vi "Day3-2.vi"() -> ()   [LabVIEW 2021]
uses:
  4dc82ad0-fb53-4f6a-a4e6-d2b65f196e0f.vi
  4388517f-81a0-45b3-bc94-ff78f6c9caee.vi
  9e6a0816-a0d4-4313-a200-a3b51abc5ec2.vi
panel:
  out "sum":i32
  out "Array":i32[](array[numeric])
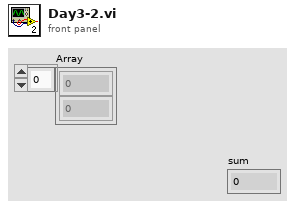
[diagram p1: front panel]
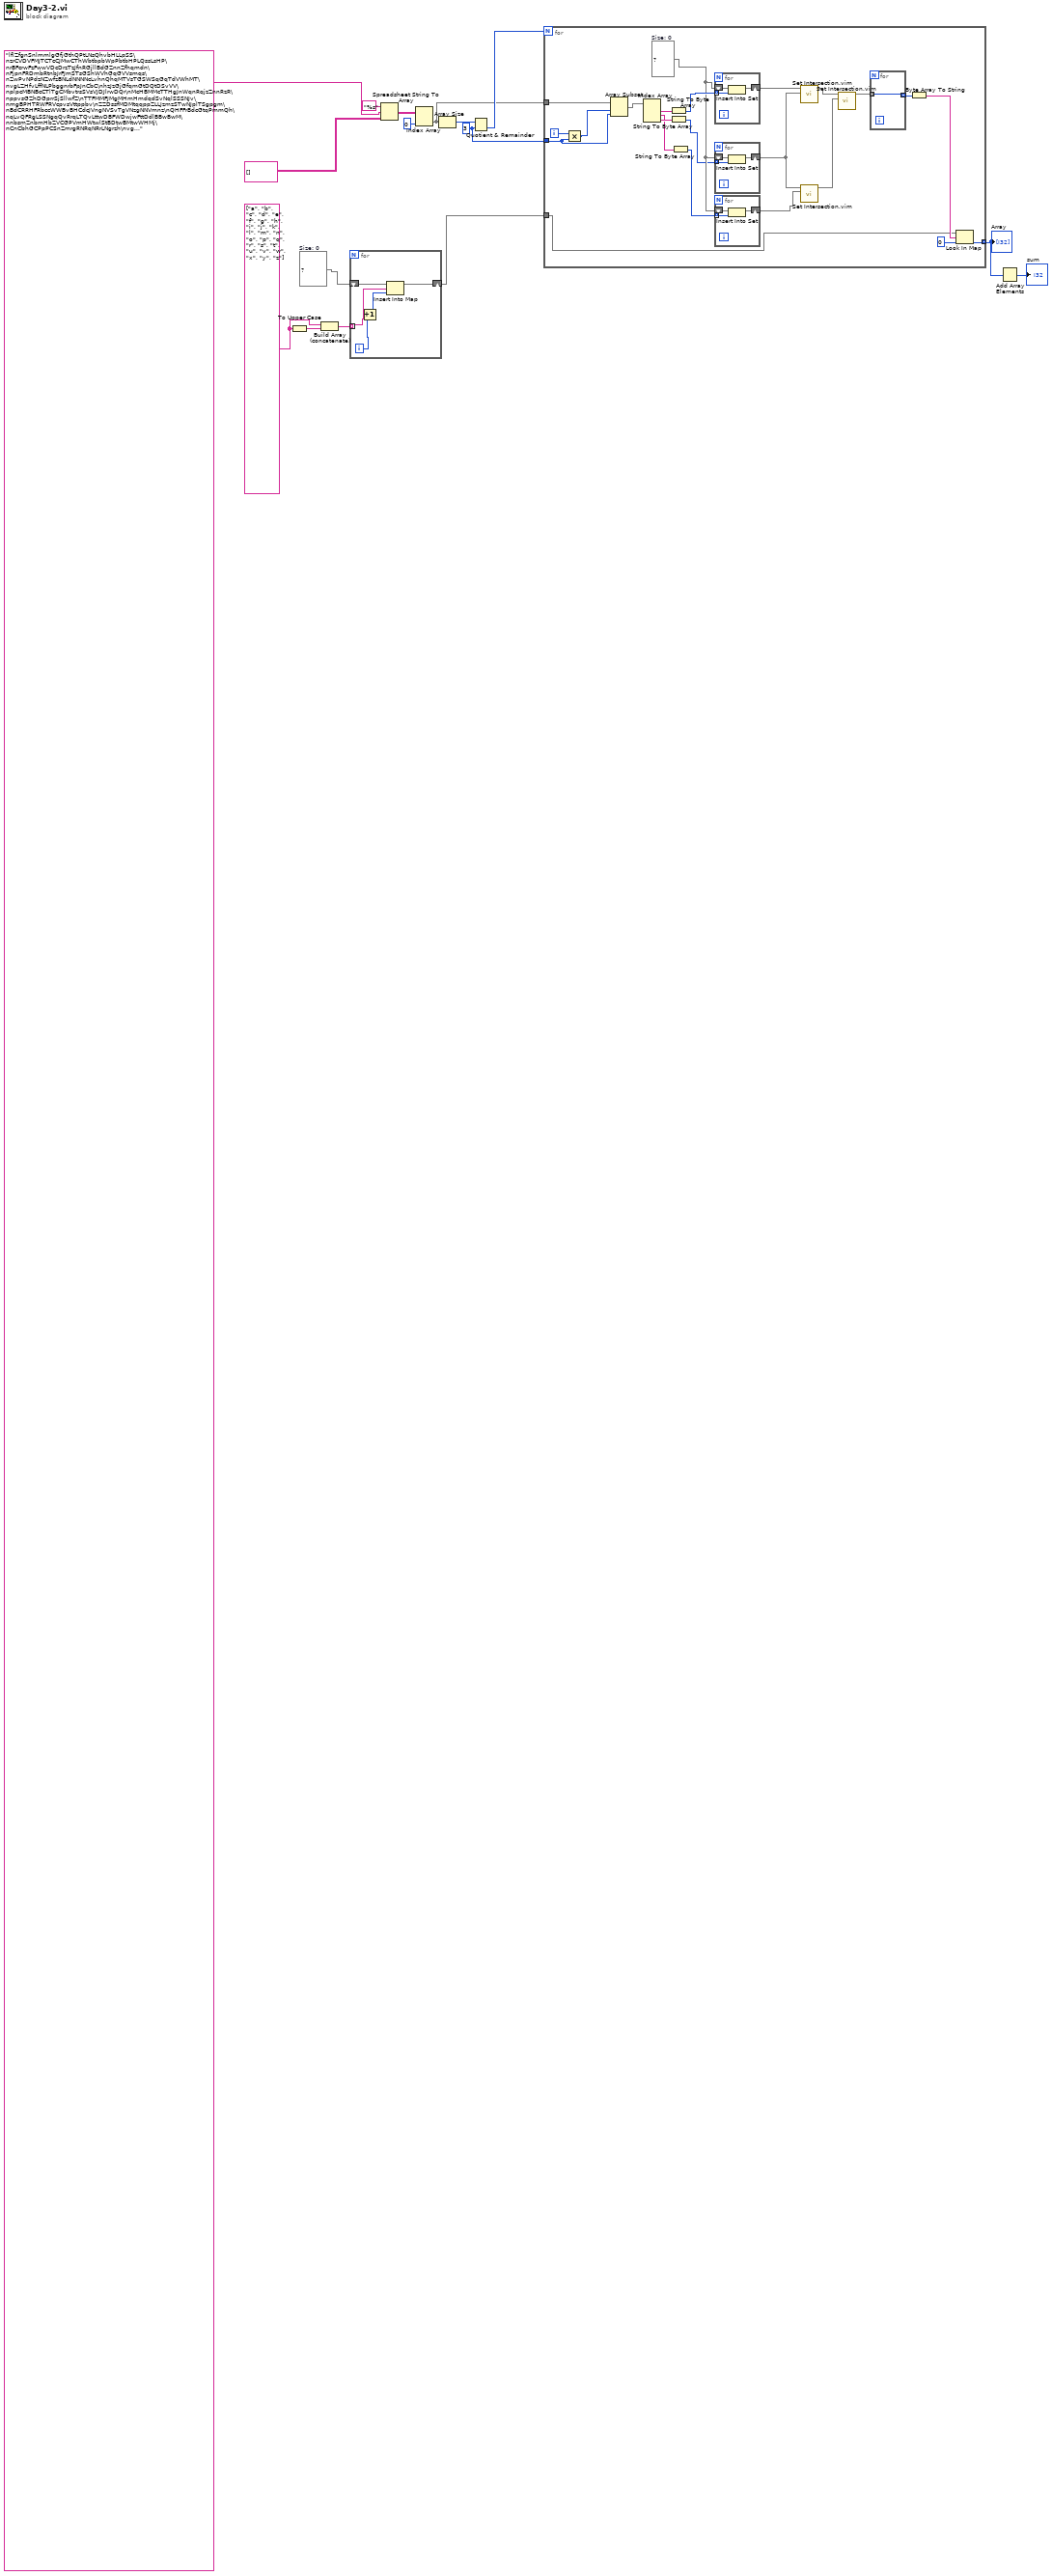
[diagram p0: block diagram]
diagram:
  w4 = 3 ("y")
  w8 = map{string, i32} {}  # Size: 0
  w10 = string[] ["a", "b", "c", "d", "e", "f", "g", "h", "i", "j", "k", "l", "m", "n", "o", "p", "q", "r", "s", "t", "u", "v", "w", "x", "y", "z"]
  n1 = To Upper Case(1:w10) -> (0:w11:string[])
  n2 = Build Array (concatenate)(w10, w11) -> (w9:string[])
  n3 = for {
    tunnel: w9 -> [w20] mode=indexing
    shift-right: [w17] -> w5
    shift-left: w8 -> [w21]
    i -> [w19]
    n4 = Increment(x=w19) -> (x+1=w18:i32)
    n5 = Insert Into Map(map in=w21, key=w20, value=w18) -> (map out=w17:map{string, i32})  [unwired: 2 out]
  }
  n6 = Spreadsheet String To Array(format string="%s", spreadsheet string="lflZfgnSnlmmlgGfjGthQPtLNsQhvbHLLpSS\nzrCVDVFMJTCTcCJMwCThWbtbpbWpPbtbHPLQssLsHP\nrBFcrwFzFwwVDcDrzTzJfnRGjllBdGZnnZfhqmdn\nFjpnFRDmbRtnbJrFJmSTsGShWVhGqGVVsmqs\nZwPvNPdzNZwfzBNLdNNNNcLvhnQhqMTVsTGSWSqGqTdVWhMT\nvgLZHfvLffNLPbggnrbFpJnCbC\nhzJzGjGfqmGtDQtDSvVV\nplpcMBNBcCTlTgCMbvtrsSVsVJDJlrwDQr\nMcHBMMcTTHgJnWqnRqjzZnnRzR\nppvsGZhDGprrSjSllwfZ\nTTFMMFJMgMHmHmdqdSvNqlSSSNJv\nmgBPHTRWFRVcpvsVttppbv\nZZDssfMDMtqqppZLLJzmzSTwNJplTSgpgm\nBdCRRHFRbccWWBvBHCdcJVngNVSvTgVNzgNNVmnz\nQHFFrBdcGtqPmmQh\nqLvQFRgLSSNgqQvRrqLTQvLttwDBFWDwjwFttDdlBBwBwM\nnbsmZnbmHbZVCGPVmHWtwlStBDtwBMtwWHMj\nCnCbhGCPpPCSnZmrgRNRqNRrLNgrzh\nvg...", array type (2D Dbl)=string[][] []) -> (array=w13:string[][])  [unwired: 1 in]
  n7 = Index Array(array=w13, index (col)=0 ("disabled index (col)")) -> (element=w3:string[])  [unwired: 1 in]
  n8 = Array Size(array=w3) -> (size(s)=w7:i32)
  n9 = Quotient & Remainder(x=w7, y=w4) -> (floor(x/y)=w6:i32)  [unwired: 1 out]
  n10 = for {
    N: w6 -> [_]
    tunnel: w5 -> [w24]
    tunnel: w4 -> [w41]
    tunnel: w3 -> [w43]
    tunnel: [w22] -> w2 mode=indexing
    i -> [w44]
    w35 = set{u8} {}  # Size: 0
    n11 = Multiply(x=w44, y=w41) -> (x*y=w42:i32)
    n12 = Array Subset(array=w43, index=w42, length=w41) -> (w40:string[])
    n13 = Index Array(array=w40) -> (element #1=w39:string, element #2=w38:string, element #3=w37:string)  [unwired: 3 in]
    n14 = String To Byte Array(string=w39) -> (unsigned byte array=w36:u8[])
    n15 = String To Byte Array(string=w38) -> (unsigned byte array=w34:u8[])
    n16 = String To Byte Array(string=w37) -> (unsigned byte array=w33:u8[])
    n17 = for {
      shift-right: [w53] -> w32
      shift-left: w35 -> [w54]
      tunnel: w36 -> [w52] mode=indexing
      n18 = Insert Into Set(10:w52, 11:w54) -> (3:w53:set{u8})  [unwired: 1 out]
    }
    n19 = for {
      shift-right: [w50] -> w31
      shift-left: w35 -> [w51]
      tunnel: w34 -> [w49] mode=indexing
      n20 = Insert Into Set(10:w49, 11:w51) -> (3:w50:set{u8})  [unwired: 1 out]
    }
    n21 = for {
      shift-right: [w47] -> w30
      shift-left: w35 -> [w48]
      tunnel: w33 -> [w46] mode=indexing
      n22 = Insert Into Set(10:w46, 11:w48) -> (3:w47:set{u8})  [unwired: 1 out]
    }
    n23 = call "Set Intersection.vim"("set 2"=w31, "set 1"=w32) -> ("intersection"=w29:set{u8})  [unwired: 9 in]
    n24 = call "Set Intersection.vim"("set 2"=w30, "set 1"=w31) -> ("intersection"=w28:set{u8})  [unwired: 9 in]
    n25 = call "Set Intersection.vim"("set 2"=w28, "set 1"=w29) -> ("intersection"=w27:set{u8})  [unwired: 9 in]
    n26 = for {
      tunnel: w27 -> [w45] mode=indexing
      tunnel: [w45] -> w26 mode=indexing
    }
    n27 = Byte Array To String(unsigned byte array=w26) -> (string=w25:string)
    n28 = Look In Map(map=w24, key=w25, default value=0) -> (value=w22:i32)  [unwired: 1 out]
  }
  "Array" <- w2
  n29 = Add Array Elements(numeric array=w2) -> (sum=→"sum":i32)
